vi "Ballard - Arinc-429 - Clear Parameters.vi"(8 "error in (no error)":errorcluster, 11 "Node Ptr":u64 format="%.0x") -> (0 "error out":errorcluster)   [LabVIEW 2019, in "Ballard Arinc-429 System Explorer.lvlib"]
uses:
  Ballard Arinc-429 System Explorer.lvlib
  Shared/Controls and Global/Global.vi
  <vilib>/NI VeriStand/Custom Device Tools/Custom Device Utility Library/NI VeriStand - Search for All Items by GUID.vi
  <vilib>/NI VeriStand/Custom Device API/Custom Device API.lvlib
  Shared/Ballard Arinc-429 Shared.lvlib
  <vilib>/NI VeriStand/Custom Device Tools/Custom Device Utility Library/Custom Device Utility Library.lvlib
panel:
  in  "Tag":string
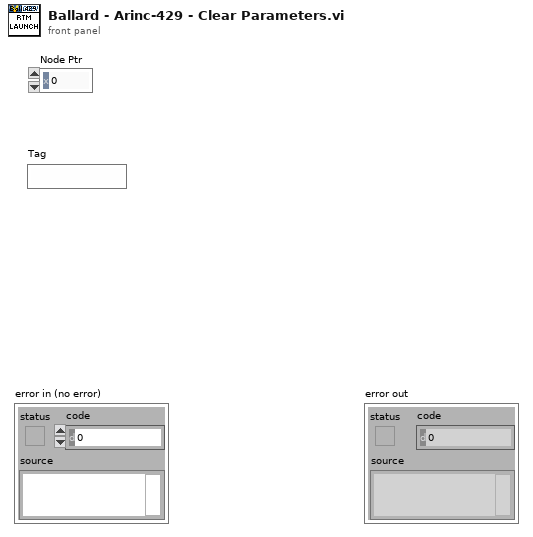
[diagram p1: front panel]
types:
  T1 = typedef "Custom Device API.lvlib/Custom Device Item Ref.ctl" = u64
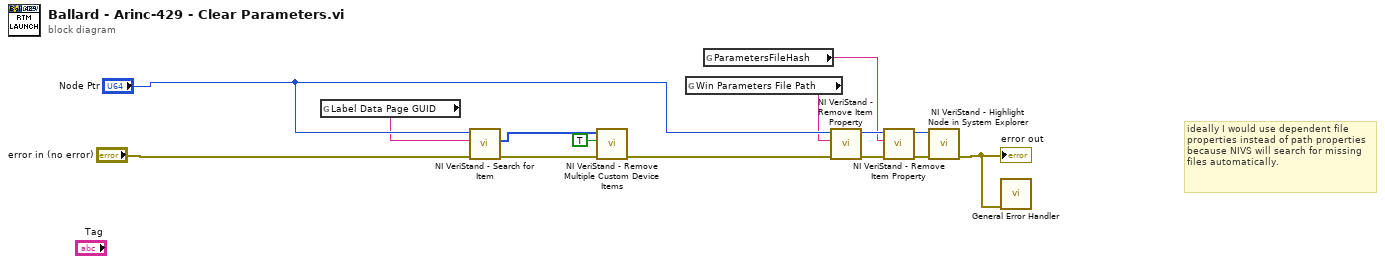
[diagram p0: block diagram]
diagram:
  # "ideally I would use dependent file properties instead of path properties because NIVS will search for missing files automatically."
  n1 = global read "Global.vi" "Label Data Page GUID"() -> (w5:string)
  n2 = call-poly <vilib>:"NI VeriStand - Search for Item.vi"("error in"="error in (no error)", "Item GUID"=w5, "Section Ref in"="Node Ptr") -> ("error out"=w4:errorcluster, "Item Refs"=w2:T1[])  [unwired: 5 in, 2 out]
  n3 = call <vilib>:"NI VeriStand - Remove Multiple Custom Device Items.vi"("error in (no error)"=w4, "Force Delete (F)"=TRUE, "Item Refs in"=w2) -> ("error out"=w1:errorcluster)  [unwired: 7 in, 1 out]
  n4 = global read "Global.vi" "Win Parameters File Path"() -> (w11:string)
  n5 = global read "Global.vi" "ParametersFileHash"() -> (w6:string)
  n6 = call <vilib>:"NI VeriStand - Remove Item Property.vi"("error in (no error)"=w1, "Property Name"=w11, "Item Ref in"="Node Ptr") -> ("error out"=w10:errorcluster, "Item Ref out"=w9:T1)  [unwired: 6 in, 1 out]
  n7 = call <vilib>:"NI VeriStand - Remove Item Property.vi"("error in (no error)"=w10, "Property Name"=w6, "Item Ref in"=w9) -> ("error out"=w8:errorcluster, "Item Ref out"=w7:T1)  [unwired: 6 in, 1 out]
  n8 = call <vilib>:"NI VeriStand - Highlight Node in System Explorer.vi"("error in (no error)"=w8, "Item Ref in"=w7) -> ("error out"=w14:errorcluster)  [unwired: 8 in, 1 out]
  "error out" <- w14
  n9 = call <vilib>:"General Error Handler.vi"("error in (no error)"=w14) -> ()  [unwired: 10 in, 5 out]
